vi "Kinematyka_jazda.vi"(6 "teta in":dbl, 7 "RAW NAPEDY 2":T1, 9 "Yo":dbl, 11 "Xo":dbl) -> (0 "po korekcie":dbl, 1 "Y":dbl, 3 "X":dbl, 4 "teta":dbl)   [LabVIEW 2015]
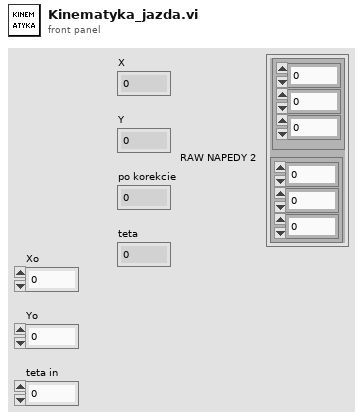
[diagram p1: front panel]
types:
  T1 = cluster{cluster{dbl, dbl, dbl}, cluster{dbl, dbl, dbl}}
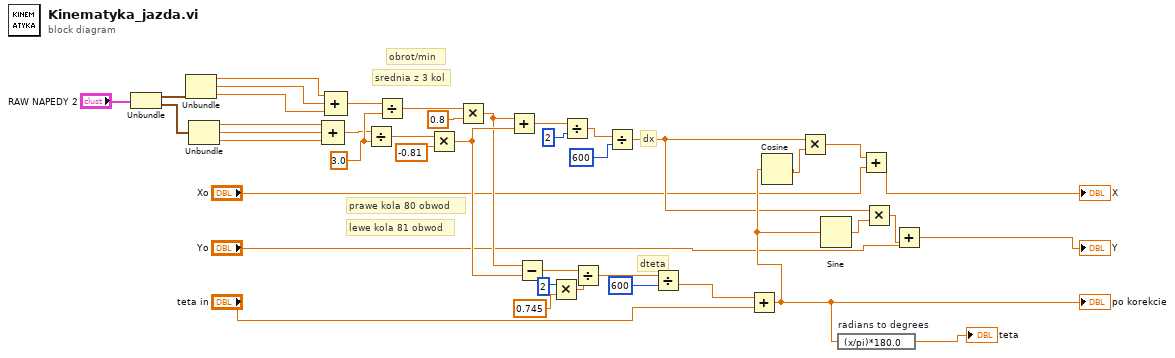
[diagram p0: block diagram]
diagram:
  w32 = 3.0
  # "srednia z 3 kol"
  # "obrot/min"
  # "dteta"
  # "dx"
  # "lewe kola 81 obwod"
  # "prawe kola 80 obwod"
  n1 = Unbundle("RAW NAPEDY 2") -> (w8:cluster{dbl, dbl, dbl}, w7:cluster{dbl, dbl, dbl})
  n2 = Unbundle(w8) -> (w3:dbl, w2:dbl, w1:dbl)
  n3 = Unbundle(w7) -> (w6:dbl, w5:dbl, w4:dbl)
  n4 = Compound Arithmetic op=ADD(w6, w5, w4) -> (w31:dbl)
  n5 = Compound Arithmetic op=ADD(w3, w2, w1) -> (w30:dbl)
  n6 = Divide(x=w31, y=w32) -> (x/y=w34:dbl)
  n7 = Divide(x=w30, y=w32) -> (x/y=w33:dbl)
  n8 = Multiply(x=w34, y=-0.81) -> (x*y=w41:dbl)
  n9 = Multiply(x=w33, y=0.8) -> (x*y=w40:dbl)
  n10 = Add(x=w40, y=w41) -> (x+y=w13:dbl)
  n11 = Subtract(x=w40, y=w41) -> (x-y=w17:dbl)
  n12 = Multiply(x=2, y=0.745) -> (x*y=w19:dbl)
  n13 = Divide(x=w13, y=2) -> (x/y=w14:dbl)
  n14 = Divide(x=w17, y=w19) -> (x/y=w35:dbl)
  n15 = Divide(x=w14, y=600) -> (x/y=w37:dbl)
  n16 = Divide(x=w35, y=600) -> (x/y=w29:dbl)
  n17 = Add(x=w29, y="teta in") -> (x+y=w38:dbl)
  "po korekcie" <- w38
  n18 = Cosine(x=w38) -> (cos(x)=w23:dbl)
  n19 = Multiply(x=w37, y=w23) -> (x*y=w24:dbl)
  n20 = Sine(x=w38) -> (sin(x)=w27:dbl)
  n21 = expression code="(x/pi)*180.0" "radians to degrees"(w38) -> (→"teta":dbl)
  n22 = Add(x=w24, y="Xo") -> (x+y=→"X":dbl)
  n23 = Multiply(x=w37, y=w27) -> (x*y=w26:dbl)
  n24 = Add(x="Yo", y=w26) -> (x+y=→"Y":dbl)
